vi "slopes_processors_list.vi"() -> ()   [LabVIEW 2020]
uses:
  SlopesPostProcessorList.lvclass
  HasoSlopes.lvclass
  HasoData.lvclass
panel:
  in  "Output Haso slopes files base name":string="Data\\data_phase_computation_processed_"
  out "Processed slopes computed and saved":bool
  out "Reference slopes loaded":bool
  out "Input slopes loaded":bool
  in  "Input Reference slopes file name":string="Data\\data_phase_computation.has"
  in  "Haso slopes files extension":string=".has"
  in  "Input Haso slopes files base name":string="Data\\data_phase_computation_"
  out "error out":errorcluster
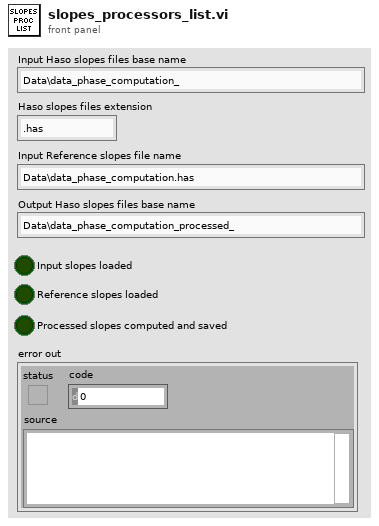
[diagram p1: front panel]
types:
  T1 = typedef "DataHaso acquisition information.ctl" = cluster{"HASO information":T2, "Acquisition information":T3, "SLOPES ENGINE information":T8, "Source wavelength (nm)":dbl, "FillPercent_%":dbl, "session_name":string}
  T2 = typedef "HASO information.ctl" = cluster{"HASO serial number":string, "HASO model":string, "Lower calibration wavelength (nm)":dbl, "Upper calibration wavelength (nm)":dbl, "Revision":i32}
  T3 = typedef "Image information.ctl" = cluster{"Image general information":T4, "Acquisition information":T5, "Number of pixels":T6, "Number of bits":T7}
  T4 = typedef "Image general information.ctl" = cluster{"Camera serial number":string, "Smearing removed":bool, "Background image removed":bool, "Time Stamp":timestamp, "Comment":string, "Camera_MAX_Level":i32}
  T5 = typedef "Image acquisition information.ctl" = cluster{"Exposure duration (us)":i32, "Exposure duration specified (us)":i32, "Gain":sgl, "Number of summed images":i32, "Trigger type":string}
  T6 = typedef "Point2D.ctl" = cluster{"X":u32, "Y":u32}
  T7 = typedef "Data alignment enum.ctl" = enum16{"8", "16", "32"}
  T8 = typedef "SlopesEngineSetup.ctl" = cluster{"Start sub-aperture":T6, "Pupil average":dbl, "AutoStartSub-aperture":bool}
  T9 = typedef "Point2Df.ctl" = cluster{"X":sgl, "Y":sgl}
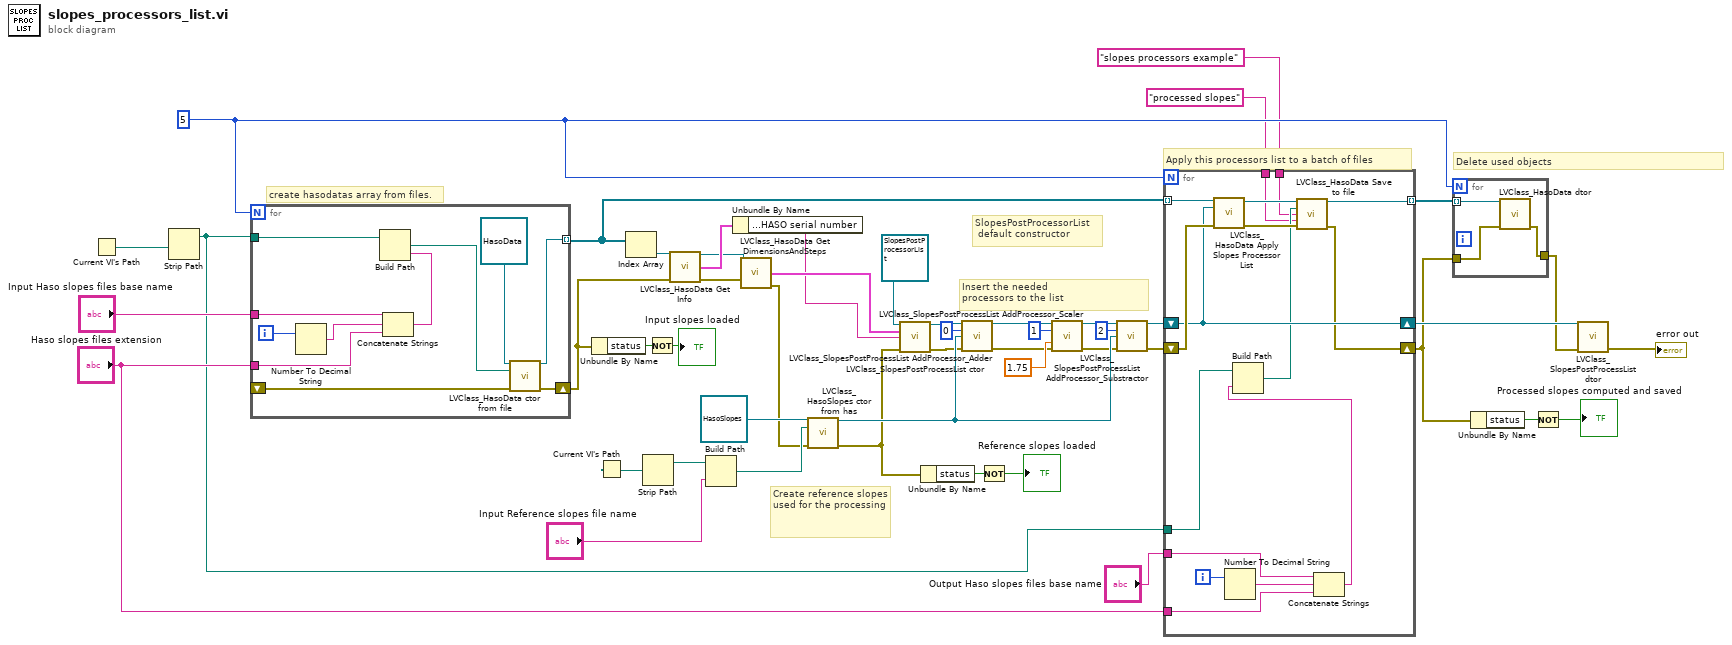
[diagram p0: block diagram]
diagram:
  w17 = 5
  # "SlopesPostProcessorList\n default constructor"
  # "Delete used objects"
  # "Apply this processors list to a batch of files"
  # "Insert the needed\nprocessors to the list"
  # "Create reference slopes used for the processing"
  # "create hasodatas array from files."
  n1 = Current VI's Path() -> (path=w27:path)
  n2 = Strip Path(path=w27) -> (stripped path=w13:path)  [unwired: 1 out]
  n3 = for {
    N: w17 -> [_]
    tunnel: w13 -> [w56]
    tunnel: [w54] -> w3 mode=indexing
    shift-right: [w52] -> w21
    shift-left: _ -> [w51]
    tunnel: "Haso slopes files extension" -> [w50]
    tunnel: "Input Haso slopes files base name" -> [w49]
    i -> [w59]
    n4 = Number To Decimal String(number=w59) -> (decimal integer string=w58:string)  [unwired: 1 in]
    n5 = Concatenate Strings(w49, w58, w50) -> (w57:string)
    n6 = Build Path(base path=w56, name or relative path=w57) -> (appended path=w55:path)
    n7 = call "LVClass_HasoData ctor from file.vi"("HasoData (const)"=refnum<class "HasoData.lvclass"> refnum ("HasoData in"), "HAS file path"=w55, "error in (no error)"=w51) -> ("HasoData (new)"=w54:refnum<class "HasoData.lvclass">, "error out"=w52:errorcluster)  [unwired: 11 in]
  }
  n8 = Unbundle By Name(w21) -> ("status"=w5:bool)
  n9 = Current VI's Path() -> (path=w25:path)
  n10 = Index Array(array=w3) -> (element=w47:refnum<class "HasoData.lvclass">)  [unwired: 1 in]
  n11 = Strip Path(path=w25) -> (stripped path=w23:path)  [unwired: 1 out]
  n12 = Not(x=w5) -> (.not. x?=→"Input slopes loaded":bool)
  n13 = call "LVClass_HasoData Get Info.vi"("HasoData in"=w47, "error in (no error)"=w21) -> ("HasoData out"=w22:refnum<class "HasoData.lvclass">, "DataHaso acquisition information"=w48:T1, "error out"=w28:errorcluster)  [unwired: 11 in]
  n14 = Build Path(base path=w23, name or relative path="Input Reference slopes file name") -> (appended path=w24:path)
  n15 = Unbundle By Name(w48) -> ("HASO information.HASO serial number"=w45:string)
  n16 = call "LVClass_HasoData Get DimensionsAndSteps.vi"("HasoData in"=w22, "error in (no error)"=w28) -> ("Dimensions"=w46:cluster{"size":T6, "steps":T9}, "error out"=w20:errorcluster)  [unwired: 11 in, 1 out]
  n17 = call "LVClass_HasoSlopes ctor from has.vi"("HasoSlopes (const)"=refnum<class "HasoSlopes.lvclass"> refnum ("HasoSlopes in"), ".has path"=w24, "error in (no error)"=w20) -> ("HasoSlopes (new)"=w34:refnum<class "HasoSlopes.lvclass">, "error out"=w18:errorcluster)  [unwired: 11 in]
  n18 = call "LVClass_SlopesPostProcessList ctor.vi"("SlopesPostProcessorList (const)"=refnum<class "SlopesPostProcessorList.lvclass"> refnum ("SlopesPostProcessorList in"), "Dimensions_um"=w46, "serial"=w45, "error in (no error)"=w18) -> ("SlopesPostProcessorList (new)"=w42:refnum<class "SlopesPostProcessorList.lvclass">, "error out"=w19:errorcluster)  [unwired: 10 in]
  n19 = Unbundle By Name(w18) -> ("status"=w9:bool)
  n20 = call "LVClass_SlopesPostProcessList AddProcessor_Adder.vi"("SlopesPostProcessorList in"=w42, "Position"=0, "HasoSlopes.lvclass"=w34, "error in (no error)"=w19) -> ("SlopesPostProcessorList out"=w40:refnum<class "SlopesPostProcessorList.lvclass">, "error out"=w37:errorcluster)  [unwired: 10 in]
  n21 = Not(x=w9) -> (.not. x?=→"Reference slopes loaded":bool)
  n22 = call "LVClass_SlopesPostProcessList AddProcessor_Scaler.vi"("SlopesPostProcessorList in"=w40, "Position"=1, "scaler"=sgl 1.75, "error in (no error)"=w37) -> ("SlopesPostProcessorList out"=w36:refnum<class "SlopesPostProcessorList.lvclass">, "error out"=w33:errorcluster)  [unwired: 10 in]
  n23 = call "LVClass_SlopesPostProcessList AddProcessor_Substractor.vi"("SlopesPostProcessorList in"=w36, "Position"=2, "HasoSlopes.lvclass"=w34, "error in (no error)"=w33) -> ("SlopesPostProcessorList out"=w32:refnum<class "SlopesPostProcessorList.lvclass">, "error out"=w31:errorcluster)  [unwired: 10 in]
  n24 = for {
    N: w17 -> [_]
    tunnel: w3 -> [w75] mode=indexing
    shift-right: [w69] -> w2
    shift-left: w31 -> [w74]
    shift-right: [w73] -> w30
    shift-left: w32 -> [w73]
    tunnel: [w70] -> w29 mode=indexing
    tunnel: "Output Haso slopes files base name" -> [w65]
    tunnel: "Haso slopes files extension" -> [w64]
    tunnel: w13 -> [w63]
    tunnel: "processed slopes" -> [w61]
    tunnel: "slopes processors example" -> [w60]
    i -> [w66]
    n25 = call "LVClass_HasoData Apply Slopes Processor List.vi"("HasoData in"=w75, "SlopesPostProcessorList"=w73, "error in (no error)"=w74) -> ("HasoData out"=w71:refnum<class "HasoData.lvclass">, "error out"=w72:errorcluster)  [unwired: 11 in]
    n26 = Number To Decimal String(number=w66) -> (decimal integer string=w67:string)  [unwired: 1 in]
    n27 = Concatenate Strings(w65, w67, w64) -> (w68:string)
    n28 = Build Path(base path=w63, name or relative path=w68) -> (appended path=w62:path)
    n29 = call "LVClass_HasoData Save to file.vi"("HasoData in"=w71, "HAS file path"=w62, "session_name"=w60, "comments"=w61, "error in (no error)"=w72) -> ("HasoData out"=w70:refnum<class "HasoData.lvclass">, "error out"=w69:errorcluster)  [unwired: 9 in]
  }
  n30 = for {
    N: w17 -> [_]
    tunnel: w29 -> [w78] mode=indexing
    tunnel: w2 -> [w77]
    tunnel: [w76] -> w10
    n31 = call "LVClass_HasoData dtor.vi"("HasoData in"=w78, "error in (no error)"=w77) -> ("error out"=w76:errorcluster)  [unwired: 12 in, 1 out]
  }
  n32 = Unbundle By Name(w2) -> ("status"=w7:bool)
  n33 = Not(x=w7) -> (.not. x?=→"Processed slopes computed and saved":bool)
  n34 = call "LVClass_SlopesPostProcessList dtor.vi"("SlopesPostProcessorList in"=w30, "error in (no error)"=w10) -> ("error out"=→"error out":errorcluster)  [unwired: 12 in, 1 out]
